vi "Fetch Data for Limits.vi"(4 "DofType":T1) -> (0 "L2 Offsets":dbl[](array[numeric]), 1 "L2 Data":dbl[](array[numeric]), 2 "L1 Offsets":dbl[](array[numeric]), 3 "L1 Data":dbl[](array[numeric]))   [LabVIEW 2013]
uses:
  Data Access Objects/Limits/DofTypes.ctl
  Dataset Source.ctl
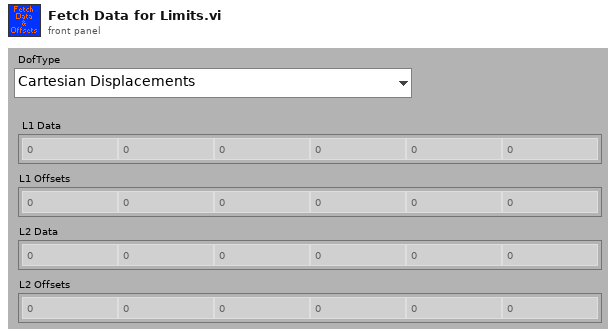
[diagram p1: front panel]
types:
  T1 = typedef "DofTypes.ctl" = enum16{"Cartesian Displacements", "Cartesian Forces & Moments", "Actuator Displacements", "Actuator Forces", "Cartesian Increments", "Actuator Increments"}
  T2 = typedef "Dataset Source.ctl" = enum16{"Continuous", "Hold", "ED", "Volts", "Offsets", "Increments"}
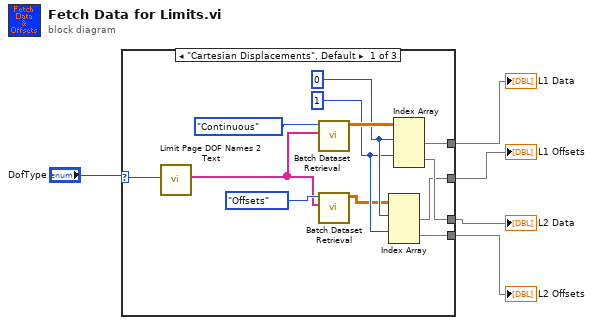
[diagram p0: block diagram]
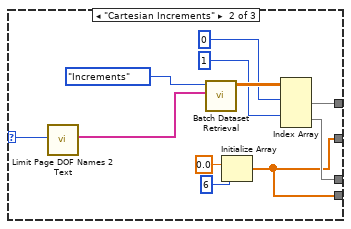
[diagram p2: hidden frame]
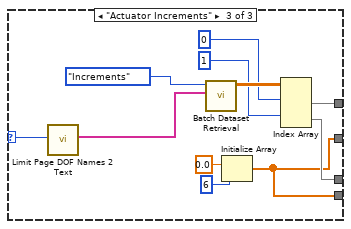
[diagram p3: hidden frame]
diagram:
  n1 = case shown="\"Cartesian Displacements\", Default" "DofType" {
    selector: "DofType" -> [w6 w22 w33]
    tunnel: [w13 w26 w37] -> w5
    tunnel: [w12 w25 w36] -> w4
    tunnel: [w8 w18 w29] -> w3
    tunnel: [w7 w18 w29] -> w2
    frame "Cartesian Displacements", Default {
      w10 = 1 ("index")
      w11 = 0 ("index")
      n2 = call "Limit Page DOF Names 2 Text.vi"("DofType"=w6) -> ("Transactions"=w15:string[])  [unwired: 10 in]
      n3 = call "Batch Dataset Retrieval.vi"("Dataset Source"=Dataset_Source."Continuous", "Transactions"=w15) -> ("Data"=w14:dbl[][])  [unwired: 7 in, 1 out]
      n4 = call "Batch Dataset Retrieval.vi"("Dataset Source"=Dataset_Source."Offsets", "Transactions"=w15) -> ("Data"=w9:dbl[][])  [unwired: 7 in, 1 out]
      n5 = Index Array(array=w9, index (row) #1=w11, index (row) #2=w10) -> (element #1=w8:dbl[], element #2=w7:dbl[])  [unwired: 2 in]
      n6 = Index Array(array=w14, index (row) #1=w11, index (row) #2=w10) -> (element #1=w13:dbl[], element #2=w12:dbl[])  [unwired: 2 in]
    }
    frame "Cartesian Increments" {
      n7 = call "Limit Page DOF Names 2 Text.vi"("DofType"=w22) -> ("Transactions"=w21:string[])  [unwired: 10 in]
      n8 = call "Batch Dataset Retrieval.vi"("Dataset Source"=Dataset_Source."Increments", "Transactions"=w21) -> ("Data"=w27:dbl[][])  [unwired: 7 in, 1 out]
      n9 = Initialize Array(0.0 ("element"), 6 ("dimension size")) -> (w18:dbl[])
      n10 = Index Array(array=w27, index (row) #1=0 ("index"), index (row) #2=1 ("index")) -> (element #1=w26:dbl[], element #2=w25:dbl[])  [unwired: 2 in]
    }
    frame "Actuator Increments" {
      n11 = call "Limit Page DOF Names 2 Text.vi"("DofType"=w33) -> ("Transactions"=w32:string[])  [unwired: 10 in]
      n12 = call "Batch Dataset Retrieval.vi"("Dataset Source"=Dataset_Source."Increments", "Transactions"=w32) -> ("Data"=w38:dbl[][])  [unwired: 7 in, 1 out]
      n13 = Initialize Array(0.0 ("element"), 6 ("dimension size")) -> (w29:dbl[])
      n14 = Index Array(array=w38, index (row) #1=0 ("index"), index (row) #2=1 ("index")) -> (element #1=w37:dbl[], element #2=w36:dbl[])  [unwired: 2 in]
    }
  }
  "L1 Data" <- w5
  "L1 Offsets" <- w3
  "L2 Data" <- w4
  "L2 Offsets" <- w2
